vi "Copy with Options.vi"(8 "error in (no error)":errorcluster, 9 "Replace Mode (Never)":enum16{"Never", "Always", "If Newer"}(ring), 10 "target path":path, 11 "source path":path) -> (0 "error out":errorcluster, 3 "new path":path)   [LabVIEW 2020]
doc: "Adds useful options to the \"Copy\" primitive. It allows to replace existing files with the options \"If Newer\", \"Never\", and \"Always\"."
panel:
  # "Copy with Options.vi\n\nAdds useful options to the \"Copy\" primitive.  It allows to replace existing files with the options \"If Newer\", \"Never\", and \"Always\".\n\nPlease visit http://www.OpenG.org to learn about the\nOpen Source LabVIEW software movement.\n\nNOTICE -- YOU MUST LEAVE THIS NOTICE IN PLACE.  PER THE TERMS OF THE LICENSE BELOW, YOU MAY SUBLICENSE THIS SOFTWARE \nIN ANY WAY THAT DOES NOT CONFLICT WITH THIS LICENSE.\n\n### BSD License (http://www.opensource.org/licenses/bsd-license.php) Begin ###\n \nCopyright (c) 2002-2006, Jim Kring <jim@jimkring.com>\n\nAll rights reserved.\n\nRedistribution and use in source and binary forms, with or without modification, are permitted provided that the following conditions are met:\n\n    * Redistributions of source code must retain the above copyright notice, this list of conditions and the following disclaimer.\n    * Redistributions in binary form must reproduce the above copyright notice, this list of conditions and the following disclaimer in the \n       documentation and/or other materials provided with the distribution.\n    * Neither the name of SciWare, James Kring, Inc., nor the names of its contributors may be used to endorse or promote products derived \n       from this software without specific prior written permission.\n\nTHIS SOFTWARE IS PROVIDED BY THE COPYRIGHT HOLDERS AND CONTRIBUTORS \"AS IS\" AND ANY EXPRESS OR IMPLIED WARRANTIES, \nINCLUDING, BUT NOT LIMITED TO, THE IMPLIED WARRANTIES OF MERCHANTABILITY AND FITNESS FOR A PARTICULAR PURPOSE ARE \nDISCLAIMED. IN NO EVENT SHALL THE COPYRIGHT OWNER OR CONTRIBUTORS BE LIABLE FOR ANY DIRECT, INDIRECT, INCIDENTAL,\n SPECIAL, EXEMPLARY, OR CONSEQUENTIAL DAMAGES (INCLUDING, BUT NOT LIMITED TO, PROCUREMENT OF SUBSTITUTE GOODS OR \nSERVICES; LOSS OF USE, DATA, OR PROFITS; OR BUSINESS INTERRUPTION) HOWEVER CAUSED AND ON ANY THEORY OF LIABILITY, \nWHETHER IN CONTRACT, STRICT LIABILITY, OR TORT (INCLUDING NEGLIGENCE OR OTHERWISE) ARISING IN ANY WAY OUT OF THE USE \nOF THIS SOFTWARE, EVEN IF ADVISED OF THE POSSIBILITY OF SUCH DAMAGE.\n\n### BSD License End ###"
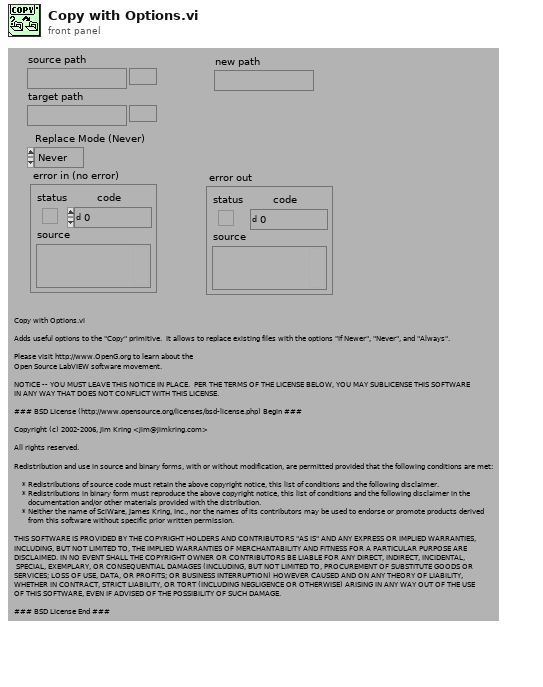
[diagram p1: front panel]
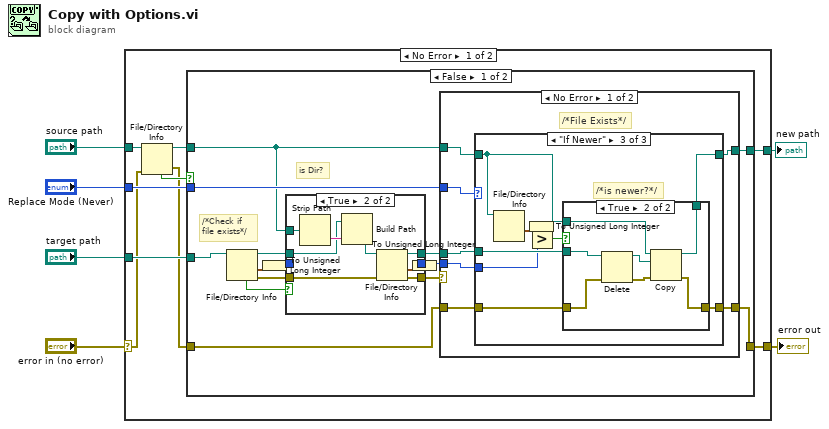
[diagram p0: block diagram]
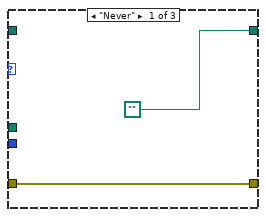
[diagram p3: hidden frame]
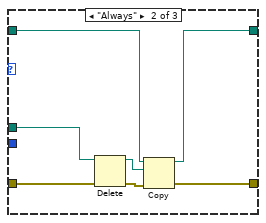
[diagram p4: hidden frame]
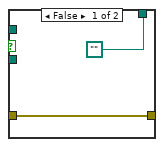
[diagram p5: hidden frame]
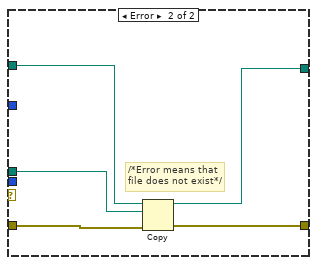
[diagram p6: hidden frame]
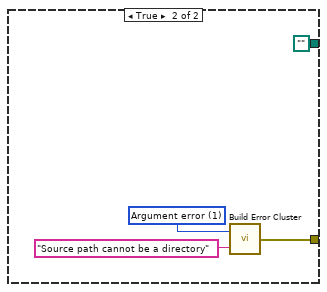
[diagram p7: hidden frame]
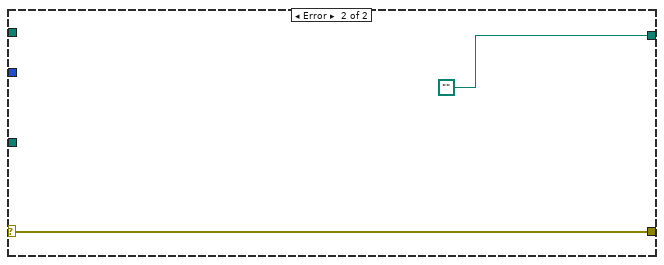
[diagram p8: hidden frame]
diagram:
  n1 = case shown="No Error" "error in (no error)" {
    selector: "error in (no error)" -> [w8 w86]
    tunnel: [w15 w86] -> w6
    tunnel: "source path" -> [w11 _]
    tunnel: "Replace Mode (Never)" -> [w14 _]
    tunnel: "target path" -> [w13 _]
    tunnel: [w12 path ""] -> w1
    frame No Error {
      n2 = File/Directory Info(path=w11, error in=w8) -> (path out=w10:path, directory=w9:bool, error out=w7:errorcluster)  [unwired: 4 out]
      n3 = case shown="False" w9 {
        tunnel: [w29 w84] -> w15
        tunnel: w14 -> [w28 _]
        tunnel: w13 -> [w27 _]
        tunnel: w7 -> [w26 _]
        tunnel: [w25 path ""] -> w12
        tunnel: w10 -> [w17 _]
        frame False {
          # "is Dir?"
          # "/*Check if file exists*/"
          n4 = File/Directory Info(path=w27) -> (path out=w23:path, directory=w24:bool, last mod=w16:timestamp, error out=w21:errorcluster)  [unwired: 1 in, 3 out]
          n5 = To Unsigned Long Integer(number=w16) -> (unsigned 32bit integer=w19:u32)
          n6 = case shown="True" w24 {
            tunnel: w17 -> [_ w41]
            tunnel: w23 -> [w30 w39]
            tunnel: [w30 w37] -> w22
            tunnel: [w32 w36] -> w20
            tunnel: w21 -> [w32 w35]
            tunnel: w19 -> [w31 _]
            tunnel: [w31 w34] -> w18
            frame False {
            }
            frame True {
              n7 = Strip Path(path=w41) -> (name=w40:string)  [unwired: 1 out]
              n8 = Build Path(base path=w39, name or relative path=w40) -> (appended path=w38:path)
              n9 = File/Directory Info(path=w38, error in=w35) -> (path out=w37:path, last mod=w33:timestamp, error out=w36:errorcluster)  [unwired: 4 out]
              n10 = To Unsigned Long Integer(number=w33) -> (unsigned 32bit integer=w34:u32)
            }
          }
          n11 = case shown="No Error" w20 {
            tunnel: w22 -> [w47 w78]
            tunnel: w18 -> [w45 _]
            tunnel: w28 -> [w48 _]
            tunnel: w17 -> [w46 w79]
            tunnel: w26 -> [w44 w77]
            tunnel: [w43 w80] -> w29
            tunnel: [w42 w76] -> w25
            frame No Error {
              # "/*File Exists*/"
              n12 = case shown="\"If Newer\"" w48 {
                tunnel: w47 -> [_ w51 w66]
                tunnel: w46 -> [_ w55 w64]
                tunnel: [w50 w54 w65] -> w43
                tunnel: w45 -> [_ _ w62]
                tunnel: w44 -> [w50 w53 w60]
                tunnel: [path "" w52 w59] -> w42
                frame "Never" {
                }
                frame "Always" {
                  n13 = Delete(path (use dialog)=w51, error in=w53) -> (deleted path=w56:path, error out=w57:errorcluster)  [unwired: 3 in, 1 out]
                  n14 = Copy(8:w57, 10:w56, 11:w55) -> (0:w54:errorcluster, 3:w52:path)  [unwired: 2 in, 1 out]
                }
                frame "If Newer" {
                  # "/*is newer?*/"
                  n15 = File/Directory Info(path=w64) -> (last mod=w58:timestamp)  [unwired: 1 in, 6 out]
                  n16 = To Unsigned Long Integer(number=w58) -> (unsigned 32bit integer=w63:u32)
                  n17 = Greater?(x=w63, y=w62) -> (0:w61:bool)
                  n18 = case shown="True" w61 {
                    tunnel: w66 -> [_ w75]
                    tunnel: [w68 w72] -> w65
                    tunnel: w64 -> [_ w71]
                    tunnel: w60 -> [w68 w70]
                    tunnel: [path "" w69] -> w59
                    frame False {
                    }
                    frame True {
                      n19 = Delete(path (use dialog)=w75, error in=w70) -> (deleted path=w73:path, error out=w74:errorcluster)  [unwired: 3 in, 1 out]
                      n20 = Copy(8:w74, 10:w73, 11:w71) -> (0:w72:errorcluster, 3:w69:path)  [unwired: 2 in, 1 out]
                    }
                  }
                }
              }
            }
            frame Error {
              # "/*Error means that file does not exist*/"
              n21 = Copy(8:w77, 10:w78, 11:w79) -> (0:w80:errorcluster, 3:w76:path)  [unwired: 2 in, 1 out]
            }
          }
        }
        frame True {
          w83 = 1 items=["No error", "Argument error", "Memory is full", "Out of zone", "End of file", "File already open", "Generic file I/O error", "File not found", "File permission error", "Disk is full", "Duplicate path", "Too many files open", "System feature not enabled", "Resource file not found", "Cannot add resource", "Resource not found", "Image not found", "Image memory error", "Pen does not exist", "Config type invalid", "Config token not found", "Config parse error", "Config memory error", "Bad external code format", "Bad external code offset", "External code not present", "Null window", "Destroy window error", "Null menu", "Print aborted", "Bad print record", "Print driver error", "Windows error during printing", "Memory error during printing", "Print dialog error", "Generic print error", "Invalid device refnum", "Device not found", "Device parameter error", "Device unit error", "Cannot open device", "Device call aborted", "Generic error", "Cancelled by user", "Object ID too low", "Object ID too high", "Object not in heap", "Unknown heap", "Unknown object (invalid DefProc)", "Unknown object (DefProc not in table)", "Message out of range", "Invalid (null) method", "Unknown message", "Manager call not supported", "Bad address", "Network operation in progress", "Network operation timed out", "Connection is busy", "Network attribute not supported", "Network error", "Address in use", "System out of memory", "Connection aborted", "Connection refused", "Not connected", "Already connected", "Connection closed", "Initialization error (interapplication manager)", "Bad occurrence", "Wait on unbound occurrence handler", "Occurrence queue overflow", "Datalog type conflict", "Unused", "Unrecognized type (interapplication manager)", "Memory corrupt", "Failed to make temporary DLL", "Old CIN version", "Drag socket not found", "Failed to load drop-object", "Failed to register OLE object", "Failed to release OLE object", "Format specifier type mismatch", "Unknown format specifier", "Too few format specifiers", "Too many format specifiers", "Scan failed", "Newer CIN version", "Error converting to variant", "Runtime menu error", "Password tampered", "Variant attribute not found", "Incompatible variant data type", "Event data is not available", "Event Store is not present", "Occurrence is not found", "Event Queue is not created", "Event info is not available", "Refnum passed is NULL", "Error retrieving Class GUID", "Error retrieving CoClass GUID", "Error retrieving TypeLib GUID.", "Bad built application magic bytes.", "Specific driver is different from the specific driver associated with the Logical Name.", "There is no session opened to the class driver.", "Max Error", "MAX - Error with config objects", "MAX - Error loading configuration", "MAX - Group not supported"]
          n22 = call "Build Error Cluster.vi"("String to Prepend to source (\"\")"="Source path cannot be a directory" ("String to Prepend to source (\"\")"), "code"=w83) -> ("error out"=w84:errorcluster)
        }
      }
    }
    frame Error {
    }
  }
  "error out" <- w6
  "new path" <- w1
